vi "Get Cell Definition.vi"(8 "error in (no error)":errorcluster, 10 "Indexes":cluster{"Row":u32, "Column":u32}, 11 "Shape Reference":refnum<data-value>) -> (0 "error out":errorcluster, 2 "Cell":refnum<class "Shape.lvclass">, 3 "Shape Reference 2":refnum<data-value>)   [LabVIEW 2017, in "LV Image Editor Framework.lvlib" / "Grid.lvclass"]
uses:
  Grid.lvclass
  Shape/Shape.lvclass
  Grid.lvclass/Grid.ctl
  Shape/Shape.lvclass/Shape.ctl
  Shape/Write Movable.vi
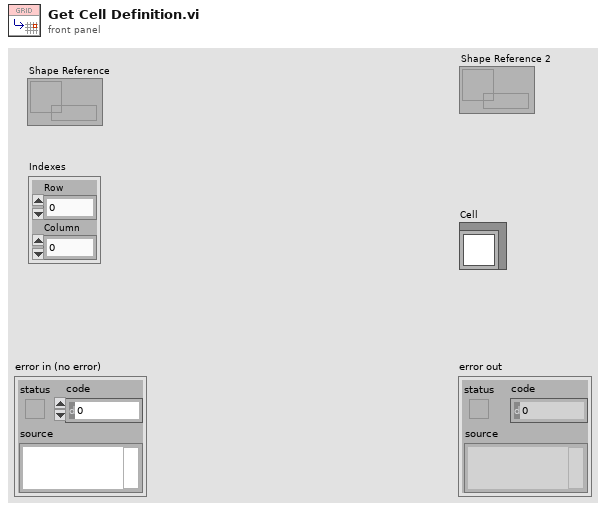
[diagram p1: front panel]
types:
  T1 = cluster{"Horizontal Step":i32, "Vertical Step":i32}
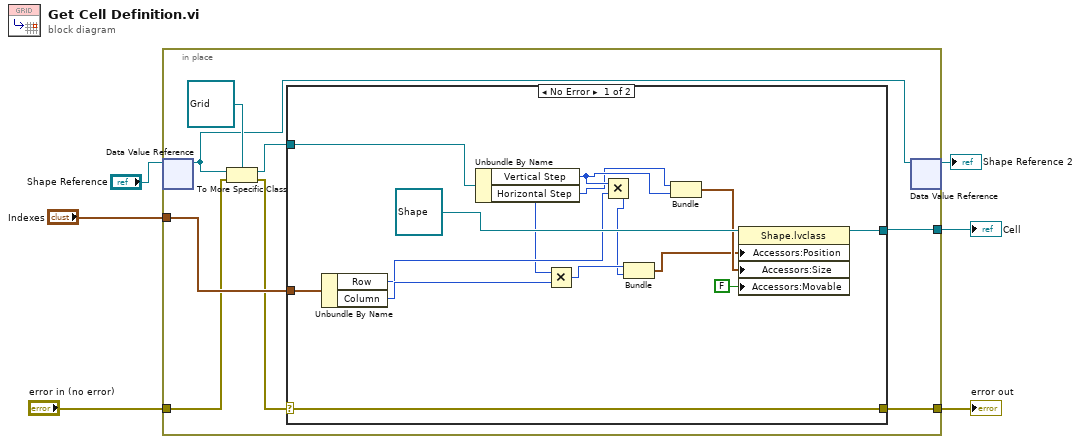
[diagram p0: block diagram]
diagram:
  n1 = in-place {
    in-place-border: "error in (no error)" -> [w8]
    in-place-border: [w14] -> w5
    in-place-border: "Indexes" -> [w13]
    in-place-border: [w11] -> w3
    n2 = in-place-dvr #1("Shape Reference") -> (w10:refnum<class "Shape.lvclass">)  [unwired: 1 out]
    n3 = To More Specific Class(target class=refnum<class "Grid.lvclass"> refnum ("Grid in"), reference=w10, error in=w8) -> (specific class reference=w7:refnum<class "Grid.lvclass">, error out=w9:errorcluster)
    n4 = case shown="No Error" w9 {
      selector: w9 -> [w28 w29]
      tunnel: [w28 w29] -> w14
      tunnel: w7 -> [w26 _]
      tunnel: w13 -> [w25 _]
      tunnel: [w17 _] -> w11
      frame No Error {
        n5 = Unbundle By Name(w25) -> ("Row"=w23:u32, "Column"=w24:u32)
        n6 = Unbundle By Name(w26) -> ("Vertical Step"=w22:i32, "Horizontal Step"=w16:i32)
        n7 = Multiply(x=w16, y=w24) -> (x*y=w20:u32)
        n8 = Multiply(x=w22, y=w23) -> (x*y=w19:u32)
        n9 = Bundle(w20, w19) -> (w18:cluster{u32, u32})  [unwired: 1 in]
        n10 = Bundle("Horizontal Step"=w16, "Vertical Step"=w22) -> (w21:T1)  [unwired: 1 in]
        n11 = property class="Shape.lvclass"(reference=refnum<class "Shape.lvclass"> refnum ("LV Image Editor Framework.lvlib:Shape.lvclass"), "Accessors:Position"=w18, "Accessors:Size"=w21, "Accessors:Movable"=FALSE ("Movable")) -> (reference out=w17:refnum<class "Shape.lvclass">)  [unwired: 1 in, 1 out]
      }
      frame Error {
      }
    }
    n12 = in-place-dvr #1(w10) -> (→"Shape Reference 2":refnum<data-value>)  [unwired: 1 out]
  }
  "error out" <- w5
  "Cell" <- w3
